vi "MeasAction.vi"(8 "error in (no error)":errorcluster caption="entrée d'erreur (pas d'erreur)", 9 "CurvePointIndex":i32, 10 "AllPointIndex":i32, 11 "InstrClassIn":refnum<class "SR400.lvclass"> caption="DNL_LabVIEW Object in") -> (0 "error out":errorcluster caption="sortie d'erreur", 2 "MeasDatOut":dbl[](array[numeric]), 3 "InstrClassOut":refnum<class "SR400.lvclass"> caption="DNL_LabVIEW Object out")   [LabVIEW 2019, in "SR400.lvclass"]
uses:
  SR400.lvclass
  C:/Programmes Labview/LabScanV1A/DevicesClass/BaseDevice/BaseDevice.lvclass
  SR400.lvclass/SR400.ctl
  <vilib>/Analysis/baseanly.llb/Mean (DBL).vi
  <vilib>/Utility/file.llb/Write To Spreadsheet File (DBL).vi
  <vilib>/Analysis/NI_AALBase.lvlib
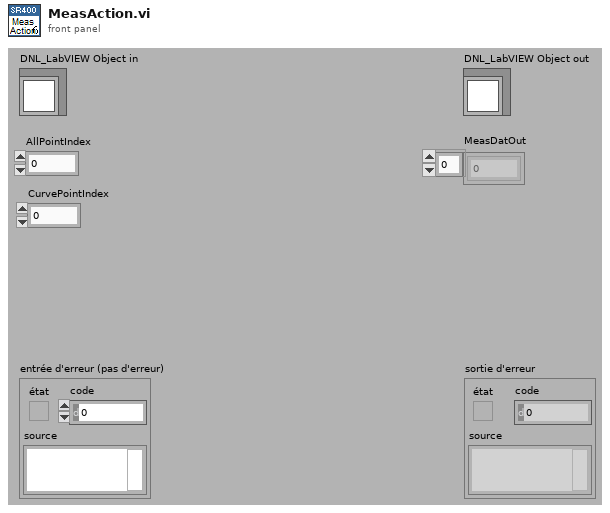
[diagram p1: front panel]
types:
  T1 = typedef "SR400.lvclass/SR400_Func.ctl" = enum16{"Read_Count (Arb)"}
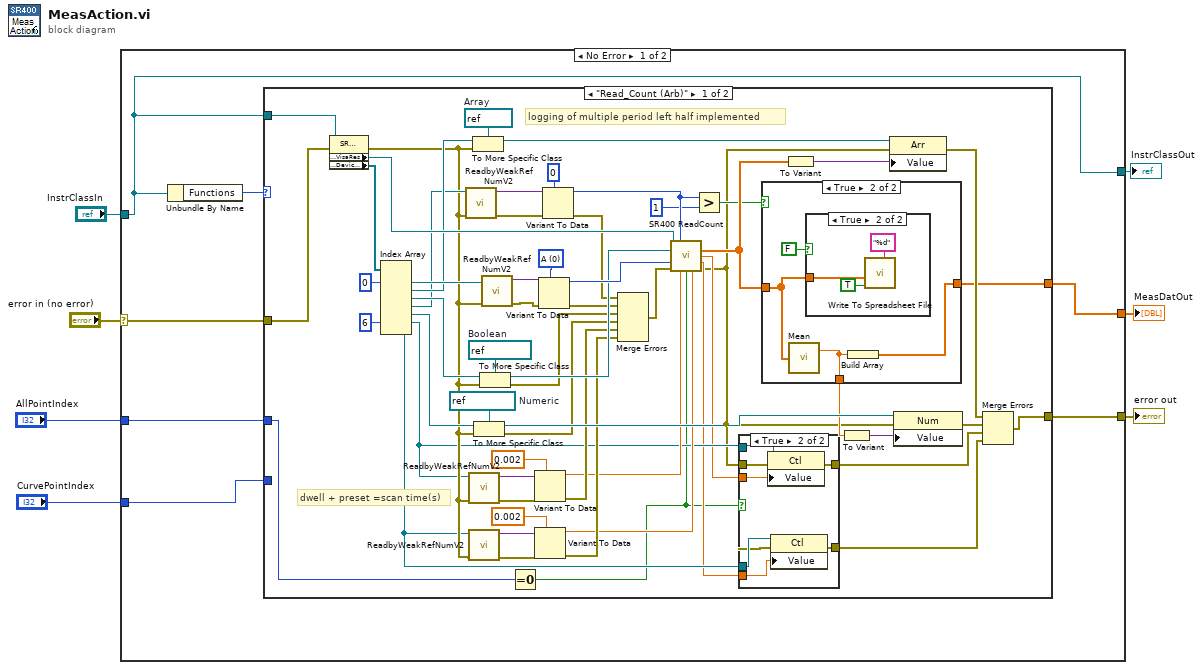
[diagram p0: block diagram]
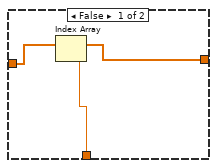
[diagram p3: hidden frame]
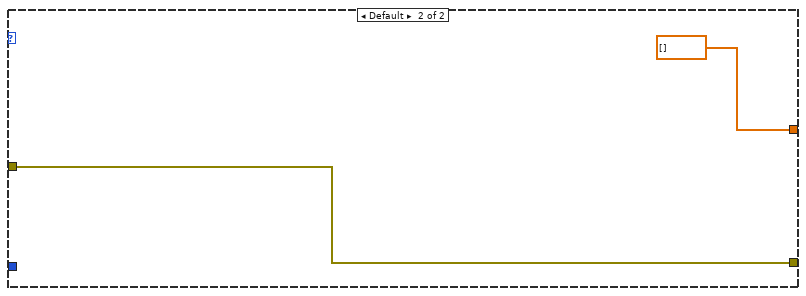
[diagram p5: hidden frame]
diagram:
  n1 = case shown="No Error" "error in (no error)" {
    selector: "error in (no error)" -> [w10 w94]
    tunnel: "InstrClassIn" -> [w8 w95]
    tunnel: [w8 w95] -> w5
    tunnel: "AllPointIndex" -> [w14 _]
    tunnel: [w13 w94] -> w3
    tunnel: [w12 _] -> w2
    tunnel: "CurvePointIndex" -> [w9 _]
    frame No Error {
      n2 = Unbundle By Name(w8) -> ("Functions"=w11:T1)
      n3 = case shown="\"Read_Count (Arb)\"" w11 {
        tunnel: w14 -> [w23 _]
        tunnel: [w49 w92] -> w13
        tunnel: [w40 dbl[] [] ("Outputs")] -> w12
        tunnel: w10 -> [w55 w92]
        tunnel: w9 -> [_ _]
        tunnel: w8 -> [w74 _]
        frame "Read_Count (Arb)" {
          w52 = refnum<vi> refnum  # Numeric
          w59 = refnum<vi> refnum  # Boolean
          w65 = refnum<vi> refnum  # Array
          w68 = u16 0 items=["A", "B", "A+B"] ("Compteur")
          # "dwell + preset =scan time(s)"
          # "logging of multiple period left half implemented"
          n4 = property class="SR400.lvclass"(reference=w74, error in=w55) -> (error out=w27:errorcluster, "Accessor:VisaRes"=w73:refnum<visa-resource-name>, "Accessor:DeviceCtrl"=w72:refnum<vi>[])  [unwired: 1 out]
          n5 = Index Array(array=w72, index #1=0 ("index"), index #6=6 ("index")) -> (element #1=w70:refnum<vi>, element #2=w66:refnum<vi>, element #3=w61:refnum<vi>, element #4=w58:refnum<vi>, element #5=w53:refnum<vi>, element #6=w22:refnum<vi>, element #7=w20:refnum<vi>)  [unwired: 5 in]
          n6 = call <userlib>:"ReadbyWeakRefNumV2.vi"("error in"=w27, "Control Ref"=w58) -> ("error out"=w54:errorcluster, "Valeur"=w57:variant)  [unwired: 8 in]
          n7 = call <userlib>:"ReadbyWeakRefNumV2.vi"("error in"=w27, "Control Ref"=w22) -> ("error out"=w32:errorcluster, "Valeur"=w34:variant)  [unwired: 8 in]
          n8 = call <userlib>:"ReadbyWeakRefNumV2.vi"("error in"=w27, "Control Ref"=w20) -> ("error out"=w30:errorcluster, "Valeur"=w29:variant)  [unwired: 8 in]
          n9 = To More Specific Class(target class=w65, reference=w66, error in=w27) -> (specific class reference=w64:refnum<vi>)  [unwired: 1 out]
          n10 = To More Specific Class(target class=w52, reference=w53, error in=w27) -> (specific class reference=w51:refnum<vi>, error out=w43:errorcluster)
          n11 = To More Specific Class(target class=w59, reference=w61, error in=w27) -> (specific class reference=w60:refnum<vi>, error out=w44:errorcluster)
          n12 = call <userlib>:"ReadbyWeakRefNumV2.vi"("error in"=w27, "Control Ref"=w70) -> ("error out"=w35:errorcluster, "Valeur"=w69:variant)  [unwired: 8 in]
          n13 = Equal To 0?(x=w23) -> (x = 0?=w15:bool)
          n14 = Variant To Data(error in=w32, type=0.002 ("Dwell time In"), Variant=w34) -> (data=w24:dbl, error out=w31:errorcluster)
          n15 = Variant To Data(error in=w30, type=0.002 ("Dwell time In"), Variant=w29) -> (data=w25:dbl, error out=w26:errorcluster)
          n16 = Variant To Data(error in=w35, type=w68, Variant=w69) -> (data=w67:u16, error out=w45:errorcluster)
          n17 = Variant To Data(error in=w54, type=0 ("Nb de période"), Variant=w57) -> (data=w39:i32, error out=w46:errorcluster)
          n18 = Merge Errors(w46, w45, w44, w43, w31, w26) -> (w47:errorcluster)
          n19 = call <userlib>:"SR400 ReadCount.vi"("VISA Port In"=w73, "Nb de période"=w39, "AcqRef"=w60, "Compteur"=w67, "error in (no error)"=w47, "Dwell time In"=w24, "Check Status"=w15, "CounterPresT In"=w25) -> ("Données"=w42:dbl[], "Dwell time"=w21:dbl, "CounterPresT"=w19:dbl, "error out"=w18:errorcluster)  [unwired: 2 in, 2 out]
          n20 = Greater?(x=w39, y=1) -> (0:w37:bool)
          n21 = case shown="True" w15 {
            tunnel: w22 -> [_ w82]
            tunnel: w21 -> [_ w81]
            tunnel: w20 -> [_ w80]
            tunnel: w19 -> [_ w79]
            tunnel: w18 -> [w75 w78]
            tunnel: [w75 w77] -> w17
            tunnel: [w75 w76] -> w16
            frame False {
            }
            frame True {
              n22 = property class="Ctl"(reference=w82, error in=w78, "Value"=w81) -> (error out=w77:errorcluster)  [unwired: 1 out]
              n23 = property class="Ctl"(reference=w80, error in=w78, "Value"=w79) -> (error out=w76:errorcluster)  [unwired: 1 out]
            }
          }
          n24 = case shown="True" w37 {
            tunnel: w42 -> [w83 w86]
            tunnel: [w84 w87] -> w41
            tunnel: [w83 w88] -> w40
            frame False {
              n25 = Index Array(array=w83) -> (element=w84:dbl)  [unwired: 1 in]
            }
            frame True {
              n26 = call-poly <vilib>:"Mean.vi"("X"=w86) -> ("mean"=w87:dbl)  [unwired: 1 out]
              n27 = case shown="True" FALSE {
                tunnel: w86 -> [_ w91]
                frame False {
                }
                frame True {
                  n28 = call-poly <vilib>:"Write To Spreadsheet File.vi"("format (%.3f)"="%d", "append to file? (new file:F)"=TRUE, "1D data"=w91) -> ()  [unwired: 5 in, 1 out]
                }
              }
              n29 = Build Array(w87) -> (w88:dbl[])
            }
          }
          n30 = To Variant(anything=w42) -> (Variant=w63:variant)
          n31 = To Variant(anything=w41) -> (Variant=w50:variant)
          n32 = property class="Arr"(reference=w64, error in=w18, "Value"=w63) -> (error out=w62:errorcluster)  [unwired: 1 out]
          n33 = property class="Num"(reference=w51, error in=w18, "Value"=w50) -> (error out=w48:errorcluster)  [unwired: 1 out]
          n34 = Merge Errors(w62, w48, w17, w16) -> (w49:errorcluster)
        }
        frame Default {
        }
      }
    }
    frame Error {
    }
  }
  "error out" <- w3
  "InstrClassOut" <- w5
  "MeasDatOut" <- w2
